vi "Find project information on disk.vi"(5 "Base folder":path, 11 "error in (no error)":errorcluster) -> (4 "Comments":string[](array[string]), 6 "Project info":T1[](array[typedef]), 8 "Project locations":path[](array[path]), 15 "error out":errorcluster)   [LabVIEW 2011]
uses:
  Project in icluster.ctl
  GUI/Job setup/Job and site cluster.ctl
  emi cndiates/List of all contrys(combo box).ctl
  GUI/Job setup/Tool registration ID.ctl
  Run Information.ctl
  <vilib>/Utility/VariantDataType/VariantType.lvlib
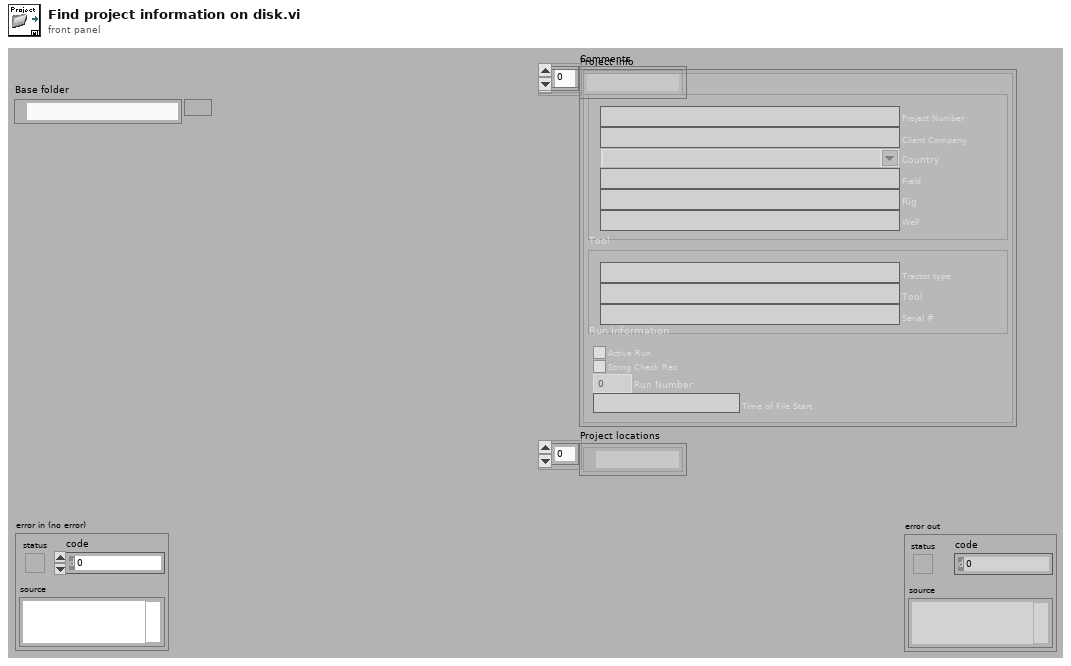
[diagram p1: front panel]
types:
  T1 = typedef "Project in icluster.ctl" = cluster{"Job and Site":T2, "Tool":T4, "Run Information":T5}
  T2 = typedef "Job and site cluster.ctl" = cluster{"Project Number":string, "Client Company":string, "Country":T3, "Field":string, "Rig":string, "Well":string}
  T3 = typedef "List of all contrys(combo box).ctl" = string
  T4 = typedef "Tool registration ID.ctl" = cluster{"Tractor type":string, "Tool":string, "Serial #":string}
  T5 = typedef "Run Information.ctl" = cluster{"Active Run":bool, "String Check Rec":bool, "Run Number":i32, "Time of File Start":string}
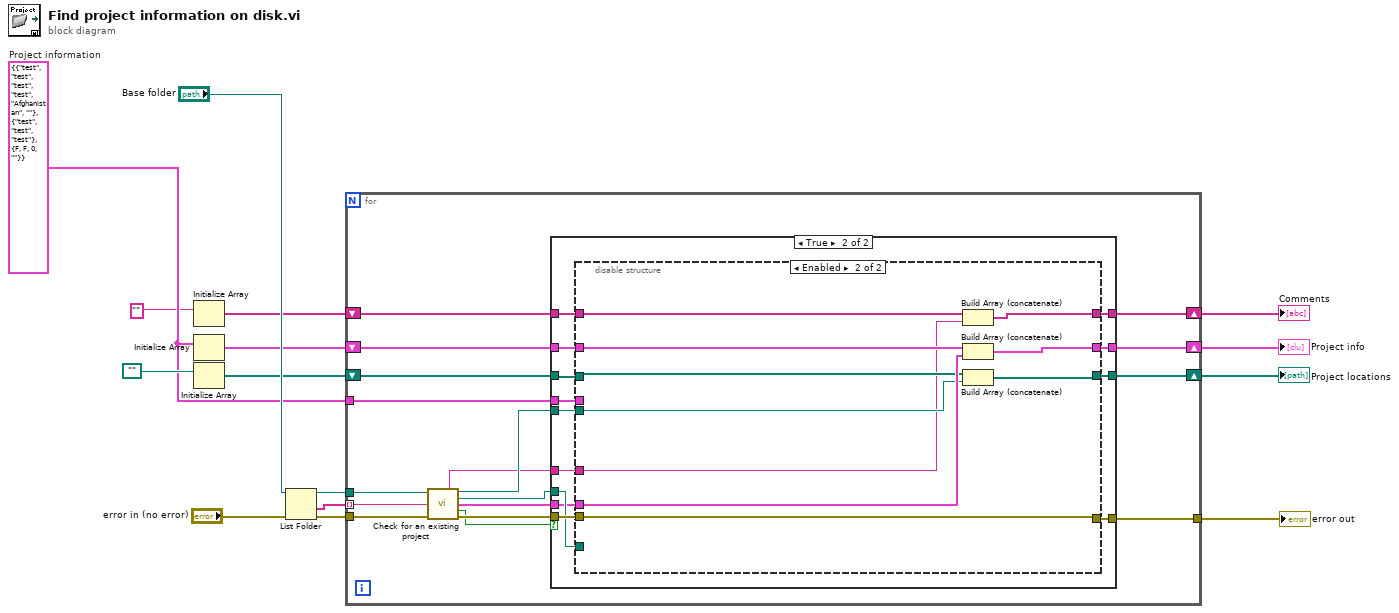
[diagram p0: block diagram]
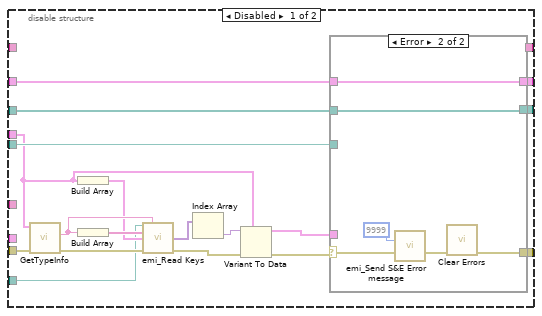
[diagram p3: hidden frame]
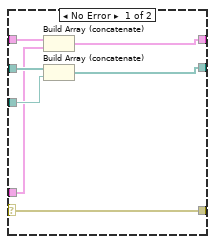
[diagram p4: hidden frame]
diagram:
  w8 = T1 {"Job and Site"={"Project Number"="test", "Client Company"="test", "Country"="test", "Field"="test", "Rig"="Afghanistan", "Well"=""}, "Tool"={"Tractor type"="test", "Tool"="test", "Serial #"="test"}, "Run Information"={"Active Run"=FALSE, "String Check Rec"=FALSE, "Run Number"=0, "Time of File Start"=""}}  # Project information
  n1 = Initialize Array("") -> (w2:string[])  [unwired: 1 in]
  n2 = Initialize Array(w8) -> (w11:T1[])  [unwired: 1 in]
  n3 = Initialize Array(path "" ("Base folder")) -> (w9:path[])  [unwired: 1 in]
  n4 = List Folder(path="Base folder", error in="error in (no error)") -> (path out=w13:path, folder names=w4:string[], error out=w12:errorcluster)  [unwired: 2 in, 1 out]
  n5 = for {
    tunnel: w4 -> [w31] mode=indexing
    tunnel: w13 -> [w32]
    tunnel: w12 -> [w30]
    shift-right: [w26] -> w6
    shift-left: w11 -> [w27]
    shift-right: [w25] -> w5
    shift-left: w9 -> [w24]
    tunnel: w8 -> [w22]
    tunnel: [w21] -> w7
    shift-right: [w16] -> w1
    shift-left: w2 -> [w17]
    n6 = call "Check for an existing project.vi"("Base folder"=w32, "Project name"=w31, "error in"=w30) -> ("Comment"=w18:string, "Project folder"=w23:path, "ini file path"=w29:path, "data"=w20:T1, "Project exists"=w19:bool, "error out"=w28:errorcluster)  [unwired: 5 in, 2 out]
    n7 = case shown="True" w19 {
      tunnel: w29 -> [_ w41]
      tunnel: w28 -> [w34 w46]
      tunnel: w27 -> [w36 w44]
      tunnel: [w36 w43] -> w26
      tunnel: [w35 w48] -> w25
      tunnel: w24 -> [w35 w49]
      tunnel: w23 -> [_ w47]
      tunnel: w22 -> [_ w45]
      tunnel: [w34 w42] -> w21
      tunnel: w20 -> [_ w40]
      tunnel: w18 -> [_ w37]
      tunnel: w17 -> [w33 w39]
      tunnel: [w33 w38] -> w16
      frame False {
      }
      frame True {
        n8 = disable-structure shown="Enabled" {
          disable-tunnel: w49 -> [w67 w87]
          disable-tunnel: [w66 w86] -> w48
          disable-tunnel: w47 -> [w65 w85]
          disable-tunnel: w46 -> [w57 w84]
          disable-tunnel: w45 -> [w56 _]
          disable-tunnel: w44 -> [w55 w90]
          disable-tunnel: [w54 w89] -> w43
          disable-tunnel: [w51 w84] -> w42
          disable-tunnel: w41 -> [w50 _]
          disable-tunnel: w40 -> [_ w88]
          disable-tunnel: w39 -> [_ w83]
          disable-tunnel: [_ w82] -> w38
          disable-tunnel: w37 -> [_ w81]
          frame Disabled {
            n9 = call <vilib>:"GetTypeInfo.vi"("error in (no error)"=w57, "Variant"=w56) -> ("error out"=w59:errorcluster, "Name"=w61:string)  [unwired: 5 in, 3 out]
            n10 = Build Array(w56) -> (w58:T1[])
            n11 = Build Array(w61) -> (w60:string[])
            n12 = call "emi_Read Keys.vi"("Ini Path(..app../config.ini)"=w50, "Section"=w61, "Key Names"=w60, "Types/Defaults"=w58, "error in (no error)"=w59) -> ("Values"=w62:variant[], "error out"=w63:errorcluster)  [unwired: 8 in, 1 out]
            n13 = Index Array(array=w62) -> (element=w64:variant)  [unwired: 1 in]
            n14 = Variant To Data(error in=w63, type=w56, Variant=w64) -> (data=w52:T1, error out=w53:errorcluster)
            n15 = case shown="Error" w53 {
              selector: w53 -> [w68 w78]
              tunnel: w67 -> [w74 w79]
              tunnel: [w73 w79] -> w66
              tunnel: w65 -> [w72 _]
              tunnel: w55 -> [w71 w80]
              tunnel: [w70 w80] -> w54
              tunnel: w52 -> [w69 _]
              tunnel: [w68 w76] -> w51
              frame No Error {
                n16 = Build Array (concatenate)(w71, w69) -> (w70:T1[])
                n17 = Build Array (concatenate)(w74, w72) -> (w73:path[])
              }
              frame Error {
                n18 = call "emi_Send S&E Error message.vi"("Loop ID in(No Loop)"=u16 9999, "error in (no error)"=w78) -> ("error out"=w77:errorcluster)  [unwired: 12 in, 1 out]
                n19 = call <vilib>:"Clear Errors.vi"("error in (no error)"=w77) -> ("error out"=w76:errorcluster)  [unwired: 6 in]
              }
            }
          }
          frame Enabled {
            n20 = Build Array (concatenate)(w83, w81) -> (w82:string[])
            n21 = Build Array (concatenate)(w90, w88) -> (w89:T1[])
            n22 = Build Array (concatenate)(w87, w85) -> (w86:path[])
          }
        }
      }
    }
  }
  "error out" <- w7
  "Project info" <- w6
  "Project locations" <- w5
  "Comments" <- w1
